vi "Data write.vi"(8 "error in (no error)":errorcluster, 9 "Parameter":string, 10 "ID":string, 11 "VISA resource name":refnum<visa-resource-name>) -> (0 "error out":errorcluster, 3 "VISA resource name out":refnum<visa-resource-name>)   [LabVIEW 2017, in "RadWag balances and scales.lvlib"]
doc: "Sends commands to balance."
uses:
  <instrlib>/Radwag Balances and Scales/Public/RadWag balances and scales.lvlib
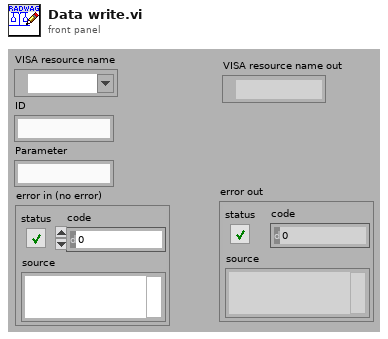
[diagram p1: front panel]
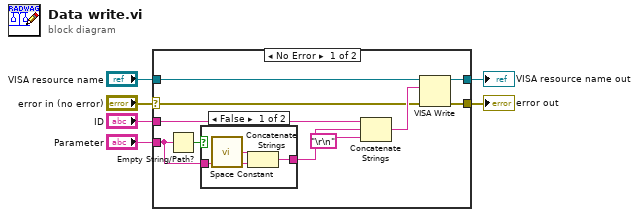
[diagram p0: block diagram]
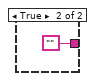
[diagram p2: hidden frame]
diagram:
  n1 = case shown="No Error" "error in (no error)" {
    selector: "error in (no error)" -> [w7 w21]
    tunnel: "VISA resource name" -> [w16 w22]
    tunnel: "ID" -> [w15 _]
    tunnel: "Parameter" -> [w11 _]
    tunnel: [w9 w22] -> w2
    tunnel: [w8 w21] -> w1
    frame No Error {
      n2 = Empty String/Path?(string/path=w11) -> (empty?=w12:bool)
      n3 = case shown="False" w12 {
        tunnel: w11 -> [w18 _]
        tunnel: [w19 ""] -> w10
        frame False {
          n4 = call <vilib>:"Space Constant.vi"() -> ("String"=w17:string)
          n5 = Concatenate Strings(w17, w18) -> (w19:string)
        }
        frame True {
        }
      }
      n6 = Concatenate Strings(w15, w10, "\r\n") -> (w14:string)
      n7 = VISA Write(VISA resource name=w16, write buffer=w14, error in (no error)=w7) -> (VISA resource name out=w9:refnum<visa-resource-name>, error out=w8:errorcluster)  [unwired: 1 out]
    }
    frame Error {
    }
  }
  "VISA resource name out" <- w2
  "error out" <- w1
